vi "Get Defer Drawing During Test.vi"(8 "error in (no error)":errorcluster) -> (0 "error out":errorcluster, 2 "Defer Drawing During Test":bool)   [LabVIEW 2017, in "Test Explorer.lvlib"]
uses:
  Test Explorer.lvlib
  Configuration/Configuration.lvlib
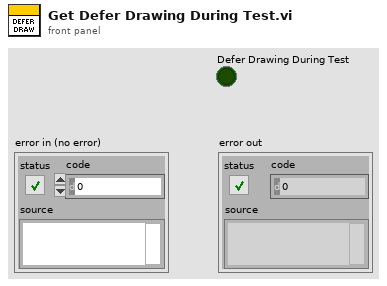
[diagram p1: front panel]
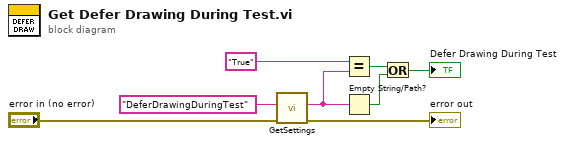
[diagram p0: block diagram]
diagram:
  n1 = call "GetSettings.vi"("error in (no error)"="error in (no error)", "Name"="DeferDrawingDuringTest") -> ("error out"=→"error out":errorcluster, "Value"=w4:string)  [unwired: 8 in]
  n2 = Equal?(x="True" ("regular expression"), y=w4) -> (x = y?=w3:bool)
  n3 = Empty String/Path?(string/path=w4) -> (empty?=w2:bool)
  n4 = Or(x=w3, y=w2) -> (x .or. y?=→"Defer Drawing During Test":bool)
